vi "Static Read.vi"(8 "error in (no error)":errorcluster, 11 "Abs_U32 Integer in":refnum<class "Abs_U32 Integer.lvclass">) -> (0 "error out":errorcluster, 2 "Value":u32, 3 "Abs_U32 Integer out":refnum<class "Abs_U32 Integer.lvclass">)   [LabVIEW 2021, in "Abs_U32 Integer.lvclass"]
uses:
  Abs_U32 Integer.lvclass
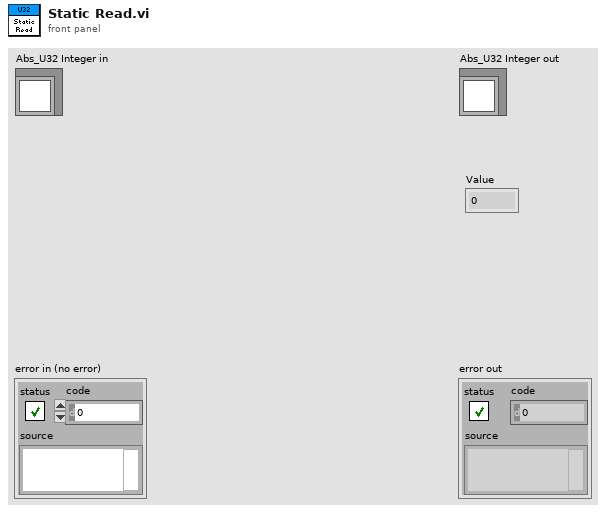
[diagram p1: front panel]
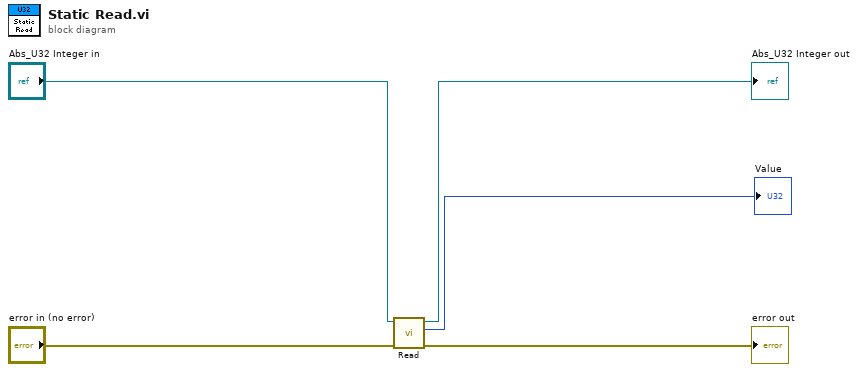
[diagram p0: block diagram]
diagram:
  n1 = call-dynamic "Read.vi"("error in (no error)"="error in (no error)", "Double Float.lvclass_340760 in"="Abs_U32 Integer in") -> ("error out"=→"error out":errorcluster, "Value"=→"Value":u32, "Double Float.lvclass_340760 out"=→"Abs_U32 Integer out":refnum<class "Abs_U32 Integer.lvclass">)  [unwired: 7 in]
